vi "Untitled 1.vi"() -> ()   [LabVIEW 2018]
panel:
  out "Time 2":u32
  out "Time":u32
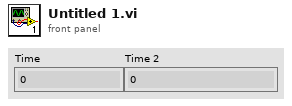
[diagram p1: front panel]
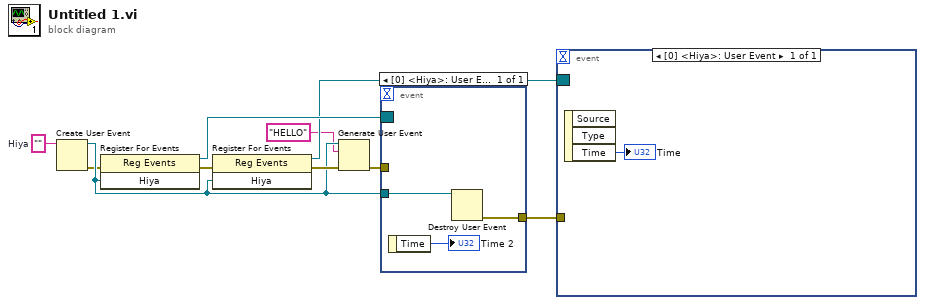
[diagram p0: block diagram]
diagram:
  w10 = ""  # Hiya
  n1 = Create User Event(user event datatype=w10) -> (user event=w4:refnum<user-event>, error out=w2:errorcluster)  [unwired: 1 in]
  n2 = register-events(error in=w2, w4) -> (reference out=w9:refnum<event-registration>, error out=w1:errorcluster)  [unwired: 1 in]
  n3 = register-events(error in=w1, w4) -> (reference out=w8:refnum<event-registration>, error out=w6:errorcluster)  [unwired: 1 in]
  n4 = Generate User Event(user event=w4, event data cluster="HELLO" ("event data"), error in=w6) -> (error out=w5:errorcluster)  [unwired: 1 in, 1 out]
  n5 = event shown="[0] <Hiya>: User Event" {
    selector: w9 -> [_]
    dyn-events: _ -> [_]
    timeout: _ -> [_]
    tunnel: w4 -> [w13]
    tunnel: [w12] -> w7
    tunnel: w5 -> [_]
    event User Event {
      n6 = event-data() -> ("Time"=→"Time 2":u32)  [unwired: 1 in]
      n7 = Destroy User Event(user event=w13) -> (error out=w12:errorcluster)  [unwired: 1 in]
    }
  }
  n8 = event shown="[0] <Hiya>: User Event" {
    selector: w8 -> [_]
    dyn-events: _ -> [_]
    timeout: _ -> [_]
    tunnel: w7 -> [_]
    event User Event {
      n9 = event-data() -> ("Time"=→"Time":u32)  [unwired: 1 in, 2 out]
    }
  }
